vi "Exemple_Preprocessing_MultiLabelBinarizer.vi"() -> ()   [LabVIEW 2020]
uses:
  Objet/6 - Datasets Transformation/6.3 - Processing Data/MultiLabelBinarizer/MultiLabelBinarizer.lvclass
panel:
  in  "y":string[][](array[string])=[["sci-fi"], ["thriller"], ["comedy"]]
  out "Data":T1
  out "error out":errorcluster
  in  "error in":errorcluster caption="entrée d'erreur"
  in  "MultiLabelBinarizer":T2
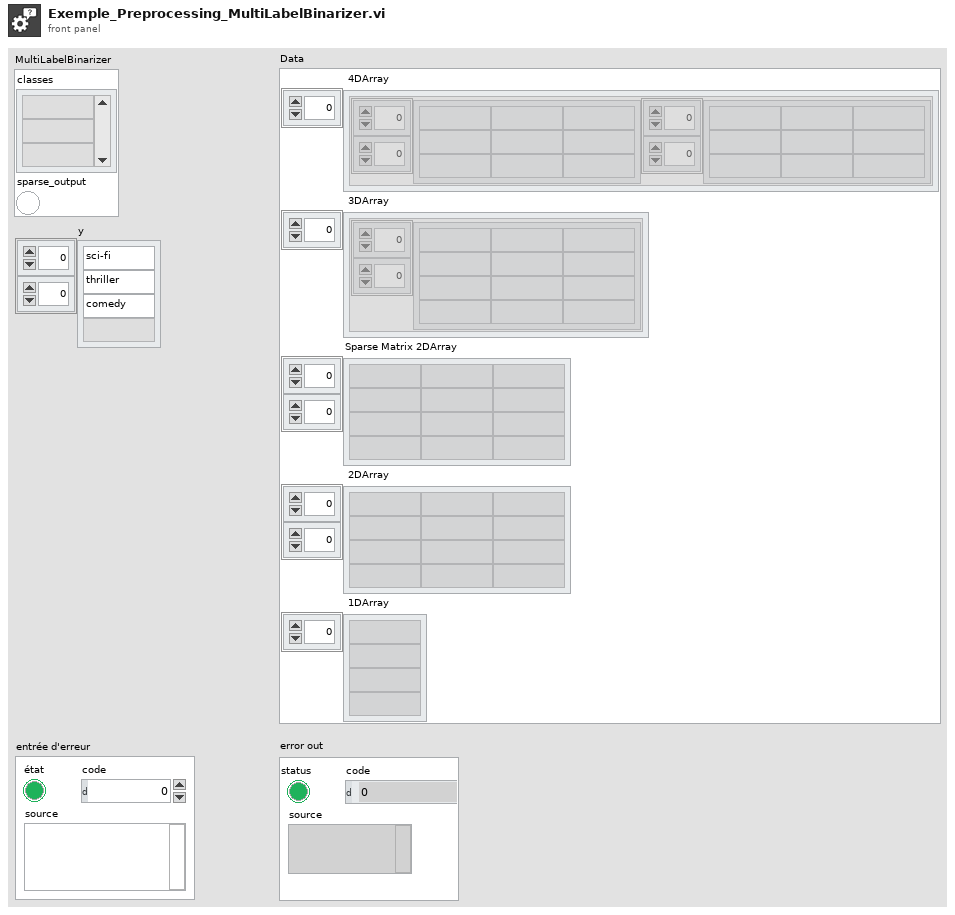
[diagram p1: front panel]
types:
  T1 = cluster{" 4DArray":cluster{"1":string[][], "2":string[][]}[], " 3DArray":cluster{"Tableau":string[][]}[], "Sparse Matrix 2DArray":string[][], " 2DArray":string[][], " 1DArray":string[]}
  T2 = cluster{"classes":string[][], "sparse_output":bool}
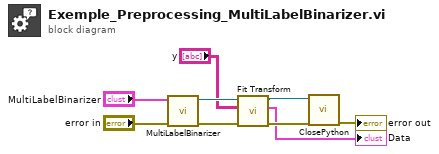
[diagram p0: block diagram]
diagram:
  n1 = call "MultiLabelBinarizer.vi"("error in (no error)"="error in", "MultiLabelBinarizer"="MultiLabelBinarizer") -> ("error out"=w5:errorcluster, "MultiLabelBinarizer.lvclass"=w6:refnum<class "MultiLabelBinarizer.lvclass">)  [unwired: 8 in]
  n2 = call-dynamic "Fit Transform.vi"("error in (no error)"=w5, "y"="y", "MultiLabelBinarizer.lvclass"=w6) -> ("error out"=w7:errorcluster, "Data"=→"Data":T1, "MultiLabelBinarizer.lvclass"=w8:refnum<class "MultiLabelBinarizer.lvclass">)  [unwired: 6 in]
  n3 = call-dynamic "ClosePython.vi"("error in (no error)"=w7, "Scikit-learn en entrée"=w8) -> ("error out"=→"error out":errorcluster)  [unwired: 8 in, 1 out]
